vi "1D Wave PDE Rendering.vi"(0 "PDE in":refnum<class "NI_PDE.lvclass">, 5 "U(t, x)":dbl[][](array[numeric]), 11 "error in (no error)":errorcluster) -> (4 "PDE out":refnum<class "NI_PDE.lvclass">, 6 "PDE Plot":dbl[][](graph), 8 "X Scale":T1, 10 "Y Scale":T1, 15 "error out":errorcluster)   [LabVIEW 2017, in "NI_PDE.lvlib"]
doc: "Renders the solution of the partial differential equation. You must manually select the polymorphic instance to use."
uses:
  <vilib>/gmath/NI_PDE.lvlib
  <vilib>/gmath/pde.llb/PDEClass/NI_PDE.lvclass
  <vilib>/Utility/miscctls.llb/LVOffsetAndMultiplierTypeDef.ctl
  <vilib>/gmath/pde.llb/DomainClass/Domain_Evolut_1D/NI_Domain_Evolut_1D.lvclass
  e:/builds/penguin/labview/branches/2017/dev/dist/vi.lib/gmath/pde.llb/DomainClass/NI_Domain.lvclass
  <vilib>/gmath/pde.llb/PDEClass/PDE_Wave_1D/NI_PDE_Wave_1D.lvclass
  e:/builds/penguin/labview/branches/2017/dev/dist/vi.lib/gmath/pde.llb/PDEClass/NI_PDE.lvclass
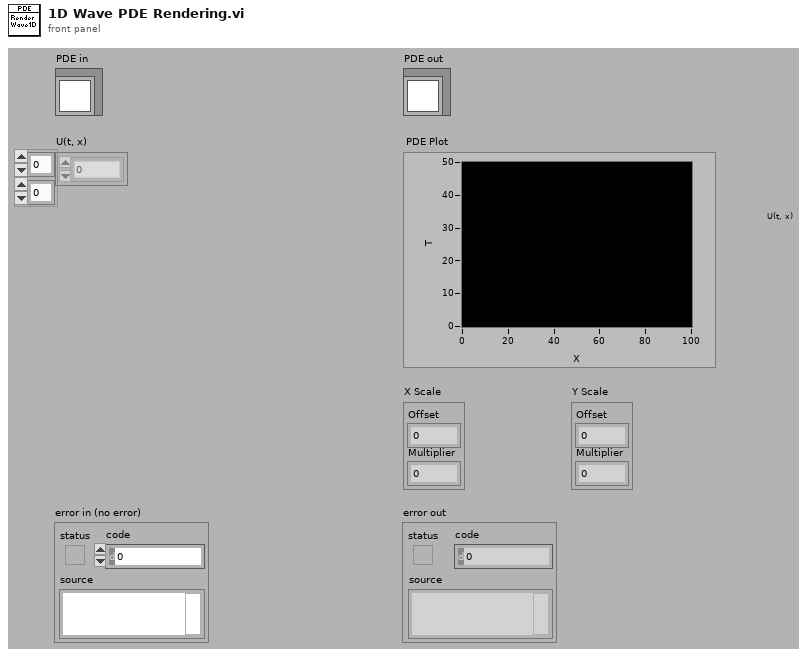
[diagram p1: front panel]
types:
  T1 = typedef "LVOffsetAndMultiplierTypeDef.ctl" = cluster{"Offset":dbl, "Multiplier":dbl}
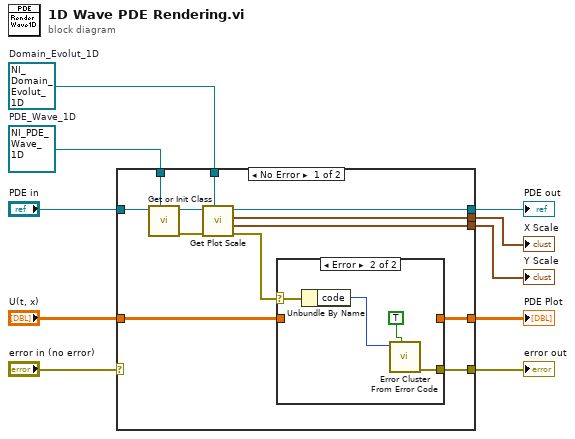
[diagram p0: block diagram]
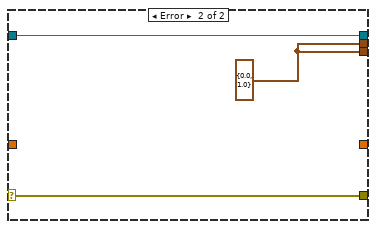
[diagram p3: hidden frame]
diagram:
  w2 = refnum<class "NI_PDE_Wave_1D.lvclass"> refnum  # PDE_Wave_1D
  w1 = refnum<class "NI_Domain_Evolut_1D.lvclass"> refnum  # Domain_Evolut_1D
  n1 = case shown="No Error" "error in (no error)" {
    selector: "error in (no error)" -> [_ w30]
    tunnel: "U(t, x)" -> [w22 _]
    tunnel: [w21 _] -> w9
    tunnel: [w16 w29] -> w8
    tunnel: "PDE in" -> [w17 w29]
    tunnel: [w14 w28] -> w6
    tunnel: [w13 w28] -> w5
    tunnel: [w20 w30] -> w4
    tunnel: w2 -> [w12 _]
    tunnel: w1 -> [w11 _]
    frame No Error {
      n2 = call <vilib>:"Get or Init Class.vi"("target PDE"=w12, "PDE in"=w17) -> ("error out"=w18:errorcluster, "PDE out"=w19:refnum<class "NI_PDE.lvclass">)  [unwired: 1 in, 7 out]
      n3 = call <vilib>:"Get Plot Scale.vi"("target Domain"=w11, "error in (no error)"=w18, "PDE in"=w19) -> ("error out"=w15:errorcluster, "Y Scale"=w13:T1, "X Scale"=w14:T1, "PDE out"=w16:refnum<class "NI_PDE.lvclass">)  [unwired: 5 out]
      n4 = case shown="Error" w15 {
        selector: w15 -> [_ w25]
        tunnel: w22 -> [w23 _]
        tunnel: [w23 _] -> w21
        tunnel: [_ w24] -> w20
        frame No Error {
        }
        frame Error {
          n5 = Unbundle By Name(w25) -> ("code"=w27:i32)
          n6 = call <vilib>:"Error Cluster From Error Code.vi"("show call chain? (False)"=TRUE, "error code (0)"=w27) -> ("error out"=w24:errorcluster)  [unwired: 1 in, 6 out]
        }
      }
    }
    frame Error {
      w28 = T1 {"Offset"=0.0, "Multiplier"=1.0} ("Offset and Multiplier")
    }
  }
  "PDE out" <- w8
  "error out" <- w4
  "PDE Plot" <- w9
  "X Scale" <- w6
  "Y Scale" <- w5
